vi "Data_SetFilePath.vi"(8 "error in (no error)":errorcluster, 10 "path":path, 11 "data in":variant) -> (0 "error out":errorcluster, 3 "data out":variant)   [LabVIEW 2017, in "FileManager.lvlib"]
uses:
  <vilib>/addons/InsightCM/Devices/Shared/Common/FileManager/FileManager.lvlib
  <vilib>/addons/InsightCM/Devices/Shared/Common/FileManager/controls/DataPropertyNames.ctl
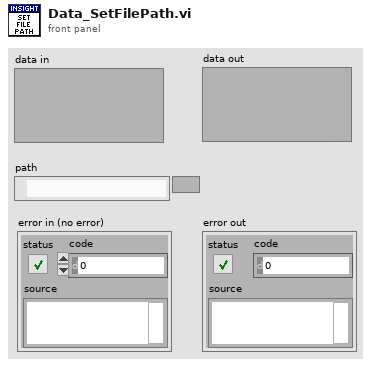
[diagram p1: front panel]
types:
  T1 = typedef "DataPropertyNames.ctl" = enum16{"Type", "EventRef", "FilePath", "DataGroup", "AcquisitionTimestamp", "StreamId", "StreamBlock", "TrendPointsOnly", "ExtraLargeFile"}
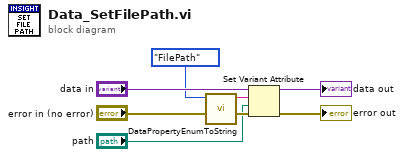
[diagram p0: block diagram]
diagram:
  n1 = call <vilib>:"DataPropertyEnumToString.vi"("property"=DataPropertyNames."FilePath" ("Names")) -> ("string"=w2:string)  [unwired: 10 in]
  n2 = Set Variant Attribute(Variant="data in", name=w2, value="path", error in="error in (no error)") -> (Variant out=→"data out":variant, error out=→"error out":errorcluster)  [unwired: 1 out]
